vi "Get Folder Shot Result as String.vi"(8 "error in (no error)":errorcluster, 11 "Folder Shot Result":T1) -> (0 "error out":errorcluster, 3 "Folder Shot Result":string)   [LabVIEW 2016, in "SLL File IO.lvlib"]
doc: "Formats the Folder Shot Results into a String."
uses:
  SLL File IO.lvlib
  _Typedefs/Folder Shot Result.ctl
  SLL String/_SubVIs/1D String Array to String.vi
  SLL String/SLL String.lvlib
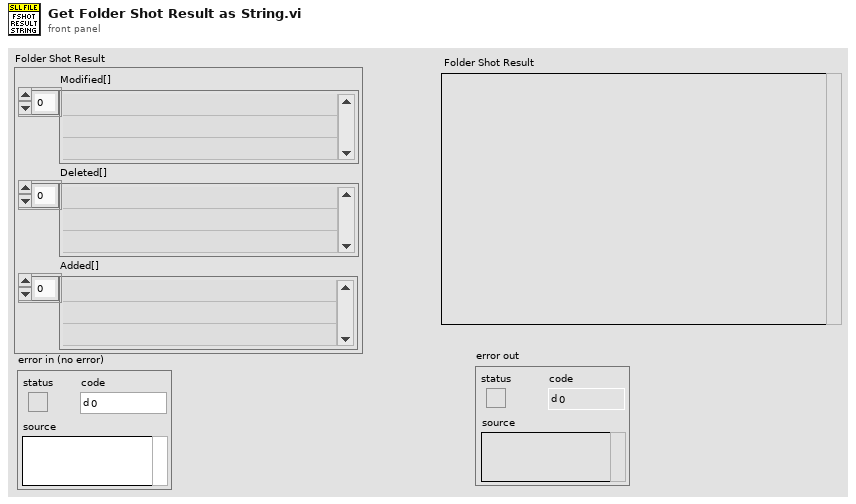
[diagram p1: front panel]
types:
  T1 = typedef "SLL File IO.lvlib/Folder Shot Result.ctl" = cluster{"Modified[]":path[], "Deleted[]":path[], "Added[]":path[]}
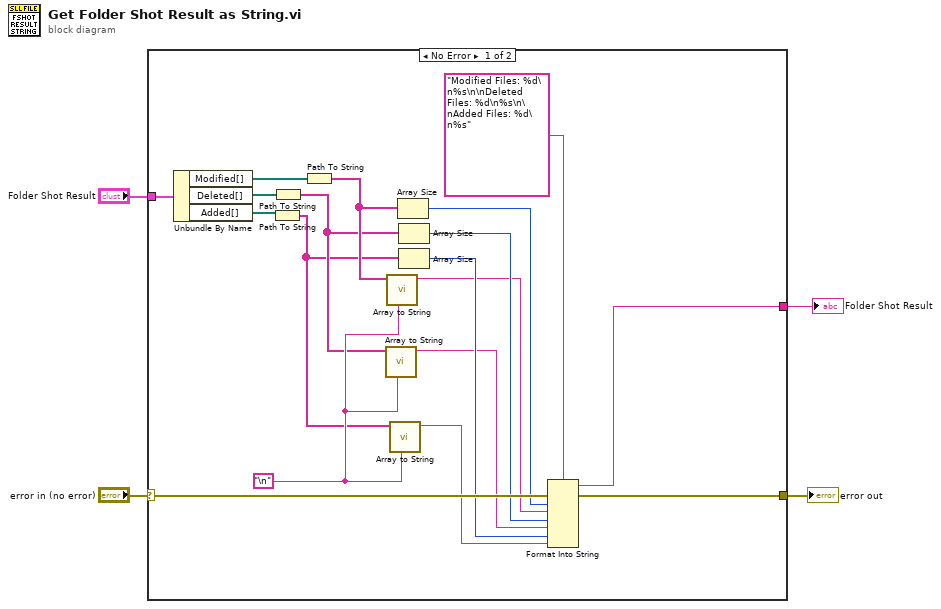
[diagram p0: block diagram]
diagram:
  n1 = case shown="No Error" "error in (no error)" {
    selector: "error in (no error)" -> [w22 w23]
    tunnel: [w16 w23] -> w3
    tunnel: "Folder Shot Result" -> [w21 _]
    tunnel: [w5 _] -> w1
    frame No Error {
      w17 = "\n"
      n2 = Unbundle By Name(w21) -> ("Modified[]"=w20:path[], "Deleted[]"=w19:path[], "Added[]"=w18:path[])
      n3 = Path To String(path=w18) -> (string=w12:string[])
      n4 = Path To String(path=w19) -> (string=w13:string[])
      n5 = Path To String(path=w20) -> (string=w14:string[])
      n6 = call-poly "Array to String.vi"("Delimiter (,)"=w17, "1D Array[]"=w13) -> ("String"=w7:string)  [unwired: 8 in, 1 out]
      n7 = call-poly "Array to String.vi"("Delimiter (,)"=w17, "1D Array[]"=w14) -> ("String"=w8:string)  [unwired: 8 in, 1 out]
      n8 = call-poly "Array to String.vi"("Delimiter (,)"=w17, "1D Array[]"=w12) -> ("String"=w6:string)  [unwired: 8 in, 1 out]
      n9 = Array Size(array=w14) -> (size(s)=w11:i32)
      n10 = Array Size(array=w13) -> (size(s)=w10:i32)
      n11 = Array Size(array=w12) -> (size(s)=w9:i32)
      n12 = Format Into String(format string="Modified Files: %d\n%s\n\nDeleted Files: %d\n%s\n\nAdded Files: %d\n%s", error in=w22, w11, w8, w10, w7, w9, w6) -> (resulting string=w5:string, error out=w16:errorcluster)  [unwired: 1 in]
    }
    frame Error {
    }
  }
  "error out" <- w3
  "Folder Shot Result" <- w1
